vi "LVClass_HasoEngine Compute Internal slopes.vi"(0 "HasoEngine in":refnum<class "HasoEngine.lvclass">, 7 "Image.lvclass":refnum<class "Image.lvclass">, 9 "learn_from_trimmer":bool, 11 "error in (no error)":errorcluster) -> (4 "HasoEngine out":refnum<class "HasoEngine.lvclass">, 6 "HasoSlopes (dup)":refnum<class "HasoSlopes.lvclass">, 8 "Image (dup)":refnum<class "Image.lvclass">, 14 "trimmer_quality":sgl, 15 "error out":errorcluster)   [LabVIEW 2020, in "HasoEngine.lvclass"]
doc: "Compute HasoSlopes. Please check that computation preferences have been set,\nand alignment step is completed.\n\n--------------------------------------------------------------------------------\n\n<B>HasoEngineIn </B> : HasoEngine object.\n<B>HasoEngineOut </B> : HasoEngine object.\n<B>HasoSlopes </B> : Computed Hasoslopes.\n<B>image </B> : Input image object.\n<B>align_from_trimmer </B> : If True, a possible mis-alignement is corrected by correlating the observed\n high-frequency aberrations. with a pre-calibrated map (trimmer). \n WARNING : The results may be distorted if the analyzed wavefront presents\n high-frequency aberrations or if the illuminated surface area on the sensor\n is too small (< 30%).\n<B>trimmer_quality </B> : If align_from_trimmer is true, correlation factor between the observed high-\n frequency aberrations and the pre-calibrated map.\n<B>ErrorIn </B> : Error\n<B>ErrorOut </B> : Error\n\n--------------------------------------------------------------------------------"
uses:
  HasoEngine.lvclass
  Image.lvclass
  HasoSlopes.lvclass
  HasoEngine.lvclass/HasoEngine.ctl
  LVClass_Image read Image Compat ptr.vi
  LVClass_HasoSlopes Read HasoSlopes _ property.vi
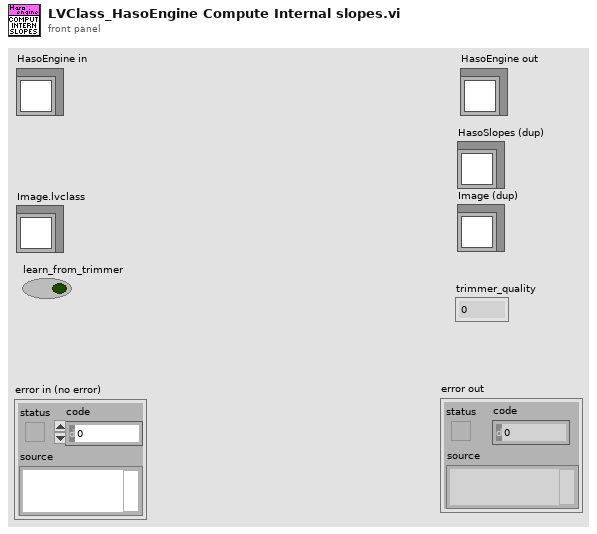
[diagram p1: front panel]
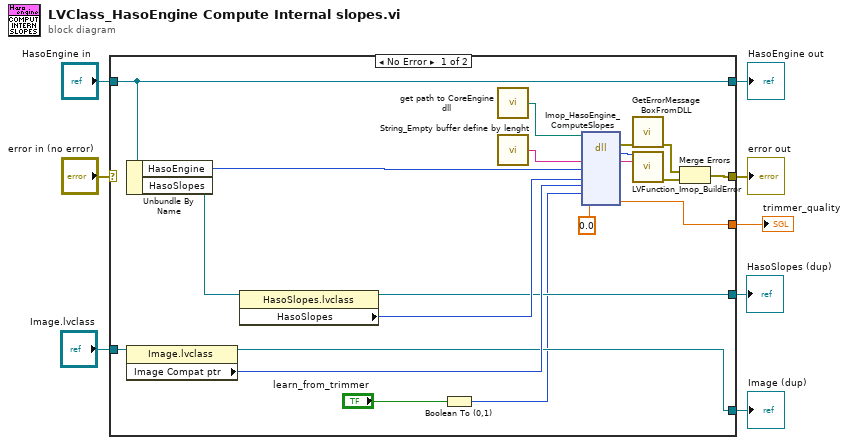
[diagram p0: block diagram]
diagram:
  n1 = case shown="No Error" "error in (no error)" {
    selector: "error in (no error)" -> [_ w30]
    tunnel: "HasoEngine in" -> [w15 w31]
    tunnel: [w15 w31] -> w5
    tunnel: [w10 w30] -> w6
    tunnel: "Image.lvclass" -> [w23 w29]
    tunnel: [w19 _] -> w3
    tunnel: [w18 w29] -> w2
    tunnel: [w9 _] -> w1
    frame No Error {
      n2 = Unbundle By Name(w15) -> ("HasoEngine"=w14:i32, "HasoSlopes"=w13:refnum<class "HasoSlopes.lvclass">)
      n3 = property class="Image.lvclass"(reference=w23) -> (reference out=w18:refnum<class "Image.lvclass">, "Image Compat ptr"=w21:i32)  [unwired: 1 in, 1 out]
      n4 = property class="HasoSlopes.lvclass"(reference=w13) -> (reference out=w19:refnum<class "HasoSlopes.lvclass">, "HasoSlopes"=w22:i32)  [unwired: 1 in, 1 out]
      n5 = Boolean To (0,1)(Boolean="learn_from_trimmer") -> (0, 1=w16:i16)
      n6 = call "get path to CoreEngine dll.vi"() -> ("path to c_interface_vc100.dll"=w25:path)  [unwired: 12 in, 3 out]
      n7 = call "String_Empty buffer define by lenght.vi"() -> ("Empty buffer"=w28:string)  [unwired: 1 in]
      n8 = dll-call lib="D:/2_trunk/Soft_haso/ImOpCoreEngine4_LV2011/DLLs/ImopEngine4_vc100.dll" fn="Imop_HasoEngine_ComputeSlopes"(path in=w25, "message"=w28, "Slopes Engine"=w14, "Data Slopes"=w22, "Image"=w21, "learn_from_trimmer"=w16, "trimmer_quality"=sgl 0.0) -> (error out=w24:errorcluster, "return type"=w26:i32, "message"=w27:string, "trimmer_quality"=w9:sgl)  [unwired: 6 in, 1 out]
      n9 = call "GetErrorMessageBoxFromDLL.vi"("error IN"=w24) -> ("error OUT"=w12:errorcluster)  [unwired: 10 in]
      n10 = call "LVFunction_Imop_BuildError.vi"("code"=w26, "String to Prepend to source (\"\")"=w27) -> ("error out"=w11:errorcluster)  [unwired: 13 in]
      n11 = Merge Errors(w12, w11) -> (w10:errorcluster)
    }
    frame Error {
    }
  }
  "error out" <- w6
  "HasoEngine out" <- w5
  "HasoSlopes (dup)" <- w3
  "Image (dup)" <- w2
  "trimmer_quality" <- w1
